vi "-8300 JSON empty--error.vi"(8 "error in":errorcluster) -> (0 "error out":errorcluster)   [LabVIEW 2025, in "Common Helpers.lvlib"]
uses:
  Common Helpers.lvlib
  Error Helpers.lvlib
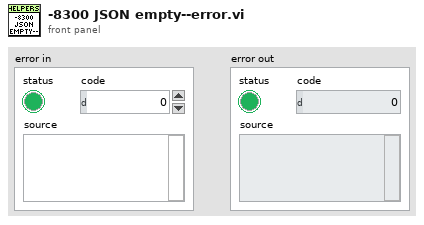
[diagram p1: front panel]
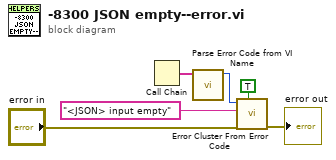
[diagram p0: block diagram]
diagram:
  n1 = Call Chain() -> (call chain=w2:string[])
  n2 = call "Parse Error Code from VI Name.vi"("Call Chain"=w2) -> ("Error Code"=w1:i32)  [unwired: 10 in]
  n3 = call <vilib>:"Error Cluster From Error Code.vi"("show call chain? (False)"=TRUE, "error in (no error)"="error in", "error message (\"\")"="<JSON> input empty" ("error message (\"\")"), "error code (0)"=w1) -> ("error out"=→"error out":errorcluster)  [unwired: 5 in]
